vi "rendszer_feldolgozása.vi"(10 "JSON  peoples":string, 11 "JSON times":string) -> ()   [LabVIEW 2015]
uses:
  <vilib>/httpClient/LabVIEWHTTPClient.lvlib
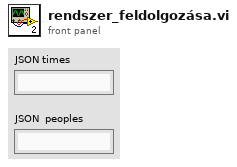
[diagram p1: front panel]
types:
  T1 = cluster{"RFID-code":string, "name":string, "user_id":dbl, "authenticated":bool}[]
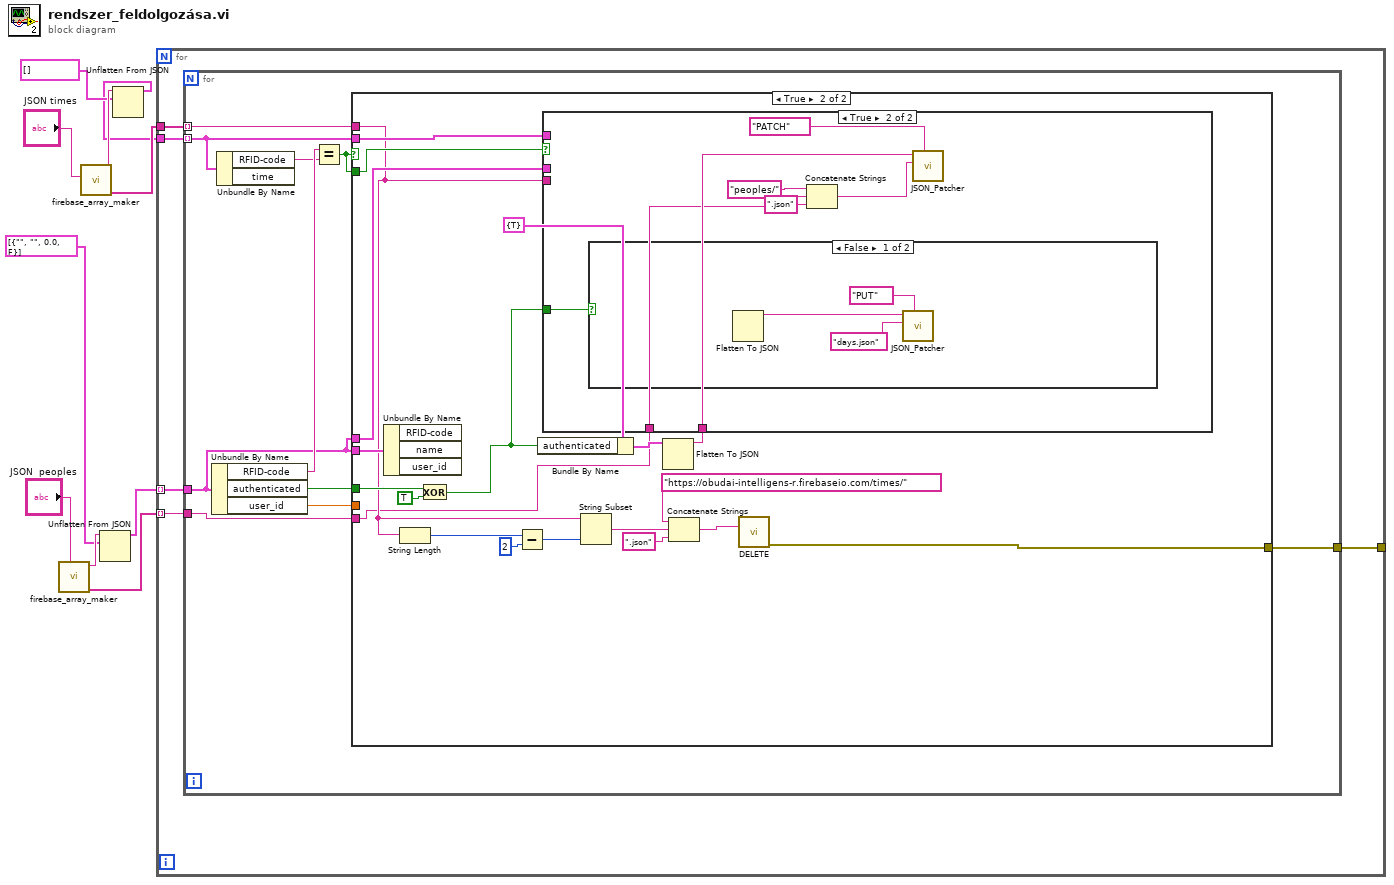
[diagram p0: block diagram]
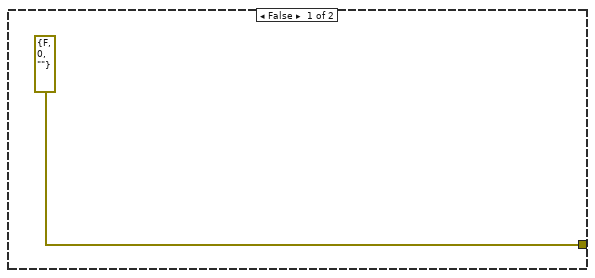
[diagram p2: hidden frame]
diagram:
  n1 = call "firebase_array_maker.vi"("be_string"="JSON  peoples") -> ("indexek_ nevei"=w8:string[], "json ki"=w3:string)  [unwired: 9 in]
  n2 = call "firebase_array_maker.vi"("be_string"="JSON times") -> ("indexek_ nevei"=w7:string[], "json ki"=w6:string)  [unwired: 9 in]
  n3 = Unflatten From JSON(JSON string=w3, type and defaults=T1 [{"RFID-code"="", "name"="", "user_id"=0.0, "authenticated"=FALSE}] ("Array")) -> (value=w2:T1)  [unwired: 5 in, 1 out]
  n4 = Unflatten From JSON(JSON string=w6, type and defaults=cluster{"RFID-code":string, "time":string}[] [] ("Array")) -> (value=w4:cluster{"RFID-code":string, "time":string}[])  [unwired: 5 in, 1 out]
  n5 = for {
    tunnel: w4 -> [w15]
    tunnel: w2 -> [w14] mode=indexing
    tunnel: w8 -> [w13] mode=indexing
    tunnel: w7 -> [w12]
    tunnel: [w11] -> _
    n6 = for {
      tunnel: w15 -> [w22] mode=indexing
      tunnel: w14 -> [w18]
      tunnel: w13 -> [w21]
      tunnel: w12 -> [w17] mode=indexing
      tunnel: [w16] -> w11
      n7 = Unbundle By Name(w18) -> ("RFID-code"=w25:string, "authenticated"=w23:bool, "user_id"=w19:dbl)
      n8 = Unbundle By Name(w22) -> ("RFID-code"=w24:string)  [unwired: 1 out]
      n9 = Equal?(x=w25, y=w24) -> (x = y?=w20:bool)
      n10 = case shown="True" w20 {
        tunnel: w23 -> [_ w36]
        tunnel: w18 -> [_ w46]
        tunnel: w22 -> [_ w45]
        tunnel: w21 -> [_ w28]
        tunnel: w20 -> [_ w44]
        tunnel: w19 -> [_ _]
        tunnel: w18 -> [_ w34]
        tunnel: w17 -> [_ w29]
        tunnel: [errorcluster {"status"=FALSE, "code"=0, "source"=""} ("error out") w33] -> w16
        frame False {
        }
        frame True {
          n11 = Unbundle By Name(w34) -> ()  [unwired: 3 out]
          n12 = String Length(string=w29) -> (length=w42:i32)
          n13 = Exclusive Or(1:TRUE ("y"), 2:w36) -> (0:w27:bool)
          n14 = Subtract(x=w42, y=2) -> (x-y=w40:i32)
          n15 = Bundle By Name(cluster=cluster{"authenticated":bool} {"authenticated"=TRUE}, "authenticated"=w27) -> (w31:cluster{"authenticated":bool})
          n16 = String Subset(string=w29, length (rest)=w40) -> (substring=w38:string)  [unwired: 1 in]
          n17 = Flatten To JSON(anything=w31) -> (JSON string=w30:string)  [unwired: 2 in, 1 out]
          n18 = case shown="True" w44 {
            tunnel: w46 -> [_ _]
            tunnel: w45 -> [_ _]
            tunnel: w29 -> [_ _]
            tunnel: w30 -> [_ w53]
            tunnel: w28 -> [_ w50]
            tunnel: w27 -> [_ w47]
            frame False {
            }
            frame True {
              n19 = case shown="False" w47 {
                frame False {
                  n20 = Flatten To JSON() -> (JSON string=w54:string)  [unwired: 3 in, 1 out]
                  n21 = call "JSON_Patcher.vi"("Küldési Mód"="PUT", "JSON utvonal"="days.json", "JSON_string"=w54) -> ()  [unwired: 8 in, 1 out]
                }
                frame True {
                }
              }
              n22 = Concatenate Strings("peoples/" ("string"), w50, ".json" ("string")) -> (w48:string)
              n23 = call "JSON_Patcher.vi"("Küldési Mód"="PATCH", "JSON utvonal"=w48, "JSON_string"=w53) -> ()  [unwired: 8 in, 1 out]
            }
          }
          n24 = Concatenate Strings("https://obudai-intelligens-r.firebaseio.com/times/" ("url"), w38, ".json" ("string")) -> (w37:string)
          n25 = call <vilib>:"DELETE.vi"("url"=w37) -> ("error out"=w33:errorcluster)  [unwired: 11 in, 3 out]
        }
      }
    }
  }
